vi "risingEdgeTest.vi"() -> ()   [LabVIEW 2014]
panel:
  in  "click":bool
  out "stop 2":bool
  in  "stop":bool
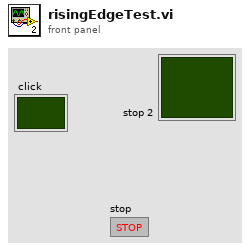
[diagram p1: front panel]
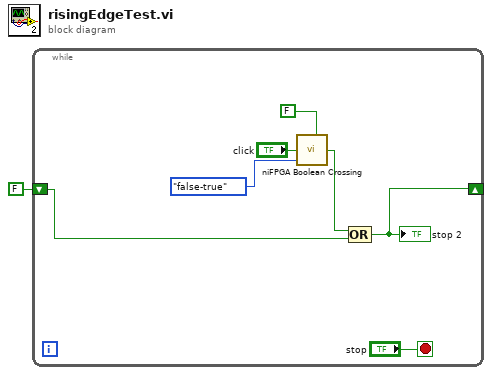
[diagram p0: block diagram]
diagram:
  n1 = while {
    shift-right: [w2] -> _
    shift-left: FALSE ("crossing") -> [w5]
    stop <- "stop" stop-if-true
    n2 = call <vilib>:"niFPGA Boolean Crossing.vi"("input"="click", "direction"=enum8{"either", "false-true", "true-false"}."false-true", "initialize"=FALSE) -> ("crossing"=w3:bool)  [unwired: 6 in]
    n3 = Compound Arithmetic op=OR(w3, w5) -> (w2:bool)
    "stop 2" <- w2
  }
